vi "TL_convert_TDMS_array_into_cluster.vi"(2 "TDMS setpoint array":dbl[][](array[numeric]), 3 "TDMS array":dbl[][](array[numeric])) -> (0 "TL - setpoint cluster":T1, 1 "TL cluster":T2={"405"=0.0, "488"=0.0, "561"=0.0, "641"=0.0, "BF "=0.0, "405 setpoint"=FALSE, "488 setpoint"=FALSE, "561 setpoint"=FALSE, "641 setpoint"=FALSE, "BF setpoint"=FALSE, "N planes 405"=0, "Dz 405"=0, "N planes 488"=0, "Dz 488"=0, "N planes 561"=0, "Dz 561"=0, "N planes 641"=0, "Dz 641"=0, "N planes BF"=0, "Dz BF"=0, "Tau 405"=inf, "Tau 488"=inf, "Tau 561"=inf, "Tau 641"=inf, "Tau BF"=inf, "405 set"=FALSE, "488 set "=FALSE, "561 set"=FALSE, "641 set"=FALSE, "BF set"=FALSE} {"Tau BF" format="%#_6e"; "Tau 641" format="%#_6e"; "Tau 561" format="%#_6e"; "Tau 488" format="%#_6e"; "Tau 405" format="%#_6e"; "641" min=0.0 max=100.0 step=0.1 scale=0.0..100.0; "561" min=0.0 max=100.0 step=0.1 scale=0.0..100.0; "405" min=0.0 max=100.0 step=0.1 scale=0.0..100.0; "488" min=0.0 max=100.0 step=0.1 scale=0.0..100.0; "BF" min=0.0 max=100.0 step=0.1 scale=0.0..100.0})   [LabVIEW 2015]
uses:
  CONTROLS/Time_lapse_parameters.ctl
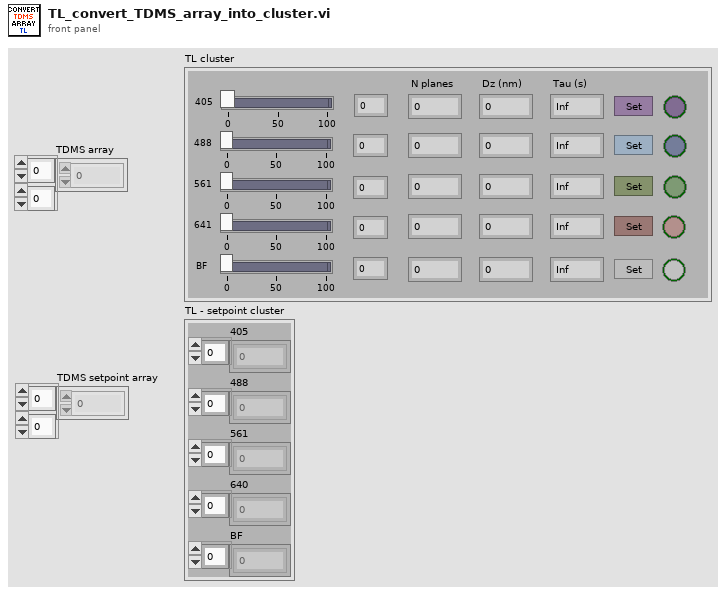
[diagram p1: front panel]
types:
  T1 = cluster{"405":dbl[], "488":dbl[], "561":dbl[], "640":dbl[], "BF":dbl[]}
  T2 = typedef "Time_lapse_parameters.ctl" = cluster{"405":dbl, "488":dbl, "561":dbl, "641":dbl, "BF ":dbl, "405 setpoint":bool, "488 setpoint":bool, "561 setpoint":bool, "641 setpoint":bool, "BF setpoint":bool, "N planes 405":i32, "Dz 405":i32, "N planes 488":i32, "Dz 488":i32, "N planes 561":i32, "Dz 561":i32, "N planes 641":i32, "Dz 641":i32, "N planes BF":i32, "Dz BF":i32, "Tau 405":dbl, "Tau 488":dbl, "Tau 561":dbl, "Tau 641":dbl, "Tau BF":dbl, "405 set":bool, "488 set ":bool, "561 set":bool, "641 set":bool, "BF set":bool}
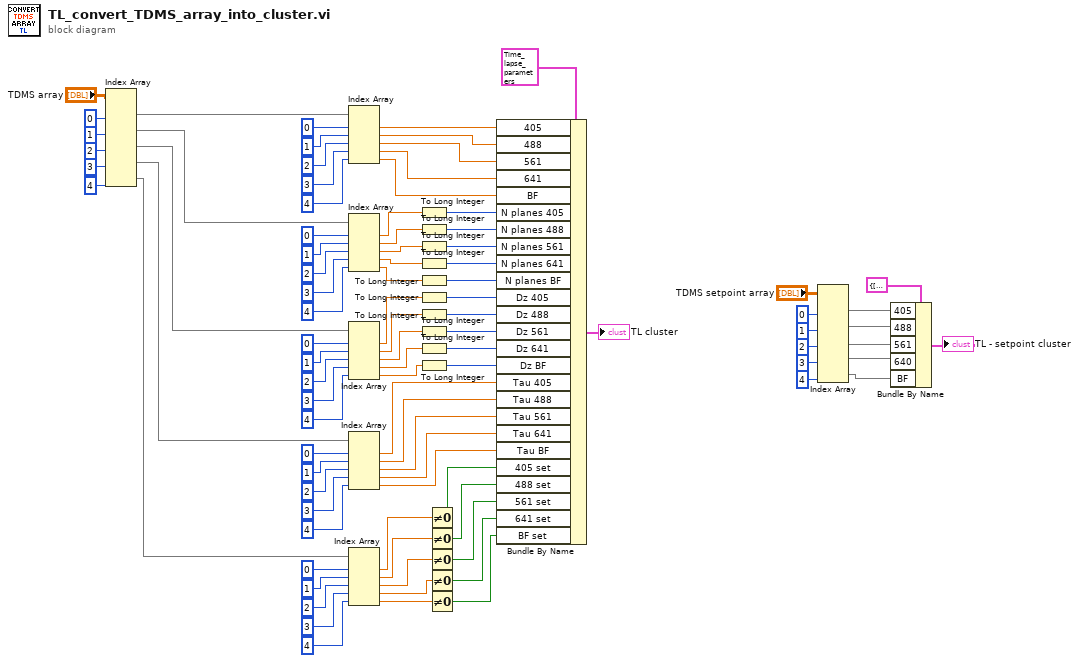
[diagram p0: block diagram]
diagram:
  n1 = Index Array(array="TDMS array", index (col) #1=0 ("disabled index (col)"), index (col) #2=1 ("index (col)"), index (col) #3=2 ("index (col)"), index (col) #4=3 ("index (col)"), index (col) #5=4 ("index (col)")) -> (element #1=w2:dbl[], element #2=w73:dbl[], element #3=w56:dbl[], element #4=w39:dbl[], element #5=w27:dbl[])  [unwired: 5 in]
  n2 = Index Array(array=w2, index #1=0 ("index"), index #2=1 ("index"), index #3=2 ("index"), index #4=3 ("index"), index #5=4 ("index")) -> (element #1=w84:dbl, element #2=w83:dbl, element #3=w82:dbl, element #4=w81:dbl, element #5=w80:dbl)
  n3 = Index Array(array=w73, index #1=0 ("index"), index #2=1 ("index"), index #3=2 ("index"), index #4=3 ("index"), index #5=4 ("index")) -> (element #1=w72:dbl, element #2=w71:dbl, element #3=w70:dbl, element #4=w69:dbl, element #5=w68:dbl)
  n4 = Index Array(array=w56, index #1=0 ("index"), index #2=1 ("index"), index #3=2 ("index"), index #4=3 ("index"), index #5=4 ("index")) -> (element #1=w50:dbl, element #2=w49:dbl, element #3=w48:dbl, element #4=w47:dbl, element #5=w46:dbl)
  n5 = Index Array(array=w39, index #1=0 ("index"), index #2=1 ("index"), index #3=2 ("index"), index #4=3 ("index"), index #5=4 ("index")) -> (element #1=w38:dbl, element #2=w37:dbl, element #3=w36:dbl, element #4=w35:dbl, element #5=w34:dbl)
  n6 = Index Array(array=w27, index #1=0 ("index"), index #2=1 ("index"), index #3=2 ("index"), index #4=3 ("index"), index #5=4 ("index")) -> (element #1=w26:dbl, element #2=w24:dbl, element #3=w22:dbl, element #4=w20:dbl, element #5=w18:dbl)
  n7 = To Long Integer(number=w72) -> (32bit integer=w67:i32)
  n8 = To Long Integer(number=w71) -> (32bit integer=w66:i32)
  n9 = To Long Integer(number=w70) -> (32bit integer=w65:i32)
  n10 = To Long Integer(number=w69) -> (32bit integer=w64:i32)
  n11 = To Long Integer(number=w68) -> (32bit integer=w63:i32)
  n12 = To Long Integer(number=w50) -> (32bit integer=w55:i32)
  n13 = To Long Integer(number=w49) -> (32bit integer=w54:i32)
  n14 = To Long Integer(number=w48) -> (32bit integer=w53:i32)
  n15 = To Long Integer(number=w47) -> (32bit integer=w52:i32)
  n16 = To Long Integer(number=w46) -> (32bit integer=w51:i32)
  n17 = Not Equal To 0?(x=w26) -> (x != 0?=w25:bool)
  n18 = Not Equal To 0?(x=w24) -> (x != 0?=w23:bool)
  n19 = Not Equal To 0?(x=w22) -> (x != 0?=w21:bool)
  n20 = Not Equal To 0?(x=w20) -> (x != 0?=w19:bool)
  n21 = Not Equal To 0?(x=w18) -> (x != 0?=w17:bool)
  n22 = Bundle By Name(cluster=T2 {"405"=0.0, "488"=0.0, "561"=0.0, "641"=0.0, "BF "=0.0, "405 setpoint"=FALSE, "488 setpoint"=FALSE, "561 setpoint"=FALSE, "641 setpoint"=FALSE, "BF setpoint"=FALSE, "N planes 405"=0, "Dz 405"=0, "N planes 488"=0, "Dz 488"=0, "N planes 561"=0, "Dz 561"=0, "N planes 641"=0, "Dz 641"=0, "N planes BF"=0, "Dz BF"=0, "Tau 405"=inf, "Tau 488"=inf, "Tau 561"=inf, "Tau 641"=inf, "Tau BF"=inf, "405 set"=FALSE, "488 set "=FALSE, "561 set"=FALSE, "641 set"=FALSE, "BF set"=FALSE} ("TL - Laser cluster"), "405"=w84, "488"=w83, "561"=w82, "641"=w81, "BF"=w80, "N planes 405"=w67, "N planes 488"=w66, "N planes 561"=w65, "N planes 641"=w64, "N planes BF"=w63, "Dz 405"=w55, "Dz 488"=w54, "Dz 561"=w53, "Dz 641"=w52, "Dz BF"=w51, "Tau 405"=w38, "Tau 488"=w37, "Tau 561"=w36, "Tau 641"=w35, "Tau BF"=w34, "405 set"=w25, "488 set"=w23, "561 set"=w21, "641 set"=w19, "BF set"=w17) -> (→"TL cluster":T2)
  n23 = Index Array(array="TDMS setpoint array", index (col) #1=0 ("disabled index (col)"), index (col) #2=1 ("index (col)"), index (col) #3=2 ("index (col)"), index (col) #4=3 ("index (col)"), index (col) #5=4 ("index (col)")) -> (element #1=w7:dbl[], element #2=w6:dbl[], element #3=w5:dbl[], element #4=w4:dbl[], element #5=w3:dbl[])  [unwired: 5 in]
  n24 = Bundle By Name(cluster=T1 {"405"=[], "488"=[], "561"=[], "640"=[], "BF"=[]} ("TL - setpoint cluster"), "405"=w7, "488"=w6, "561"=w5, "640"=w4, "BF"=w3) -> (→"TL - setpoint cluster":T1)
